vi "Main.vi"() -> ()   [LabVIEW 2017]
doc: "The myRIO Project template acquires acceleration data from the onboard accelerometer and displays the changes of acceleration values in a waveform chart."
uses:
  Y Axis Motor Cluster.ctl
  X Axis Motor Cluster.ctl
  Coords Input Cluster.ctl
  Motor Status Enum.ctl
  Encoder Cluster.ctl
  <vilib>/myRIO/Common/Instrument Driver Framework/myRIO v1.0/Encoder/typedefs/Encoder Count Direction Enum.ctl
  Motion Type Def.ctl
  <vilib>/myRIO/Instrument Drivers/Onboard IO/PWM/typedefs/PWM Reference.ctl
  <vilib>/myRIO/Common/Instrument Driver Framework/Utilities/typedefs/myRIO Generic Hardware Reference.ctl
  <vilib>/myRIO/Common/Instrument Driver Framework/Utilities/typedefs/Hardware Version Enum.ctl
  <vilib>/myRIO/Common/Instrument Driver Framework/Utilities/typedefs/myRIO v1.0 Reference.ctl
  <vilib>/myRIO/Common/Instrument Driver Framework/Utilities/typedefs/Generic FPGA Reference.ctl
  <vilib>/myRIO/Common/Instrument Driver Framework/myRIO v1.0/PWM/typedefs/PWM Channels Enum.ctl
  <vilib>/myRIO/Instrument Drivers/Onboard IO/PWM/typedefs/PWM Configuration.ctl
  <vilib>/userdefined/High Color/nirio_resource_hc.ctl
  <vilib>/myRIO/Common/Instrument Driver Framework/Utilities/vis/Is FPGA Ref Available.vi
  <vilib>/myRIO/Common/Instrument Driver Framework/myRIO v1.0/PWM/vis/myRIO v1.1 Open PWM.vi
  <vilib>/myRIO/Instrument Drivers/Onboard IO/PWM/vis/Set Duty Cycle and Frequency.vi
  <vilib>/myRIO/Common/Instrument Driver Framework/Utilities/vis/Validate Channels.vi
  <vilib>/myRIO/Common/Instrument Driver Framework/myRIO v1.0/PWM/vis/myRIO v1.0 Reserve PWM.vi
  <vilib>/myRIO/Common/Instrument Driver Framework/myRIO v1.0/UART/vis/myRIO v1.0 Close UART.vi
  <vilib>/myRIO/Common/Instrument Driver Framework/myRIO v1.0/PWM/vis/myRIO v1.0 Build MUX Configuration PWM.vi
  <vilib>/myRIO/Common/Instrument Driver Framework/myRIO v1.0/Resource Manager/vis/myRIO v1.0 Reserve Channel List.vi
  <vilib>/myRIO/Common/Instrument Driver Framework/myRIO v1.0/Resource Manager/vis/myRIO v1.0 Create Configuration List.vi
  <vilib>/myRIO/Common/Instrument Driver Framework/myRIO v1.0/Resource Manager/vis/myRIO v1.0 Reserve Channel.vi
  <vilib>/myRIO/Common/Instrument Driver Framework/myRIO v1.0/Resource Manager/vis/myRIO v1.0 Unreserve Channel.vi
  <vilib>/myRIO/Common/Instrument Driver Framework/myRIO v1.0/Resource Manager/vis/myRIO v1.0 Build Mutex Name.vi
  <vilib>/Utility/VariantDataType/GetNumericInfo.vi
  <vilib>/Utility/error.llb/Error Cluster From Error Code.vi
  <vilib>/myRIO/Common/Instrument Driver Framework/myRIO v1.0/myRIO v1.1 Open.vi
  <vilib>/myRIO/Common/Instrument Driver Framework/Utilities/vis/IO Manager.vi
  <vilib>/myRIO/Common/Instrument Driver Framework/Utilities/vis/Configuration Manager.vi
  <vilib>/myRIO/Common/Instrument Driver Framework/myRIO v1.0/Resource Manager/vis/myRIO v1.0 Configure IO.vi
  <vilib>/myRIO/Common/Instrument Driver Framework/myRIO v1.0/myRIO v1.0 Close.vi
  <vilib>/myRIO/Common/Instrument Driver Framework/myRIO v1.0/PWM/vis/myRIO v1.0 Write PWM.vi
  <vilib>/myRIO/Common/Instrument Driver Framework/Utilities/vis/FPGA Ref Manager.vi
  <vilib>/myRIO/Common/Instrument Driver Framework/myRIO v1.0/myRIO v1.0 Reset FPGA.vi
  <vilib>/myRIO/Common/Instrument Driver Framework/myRIO v1.0/IRQ/vis/myRIO v1.0 IRQ Info FGV.vi
  <vilib>/myRIO/Common/Instrument Driver Framework/myRIO v1.0/IRQ/vis/myRIO v1.0 Timer IRQ Info FGV.vi
  <vilib>/myRIO/Common/Instrument Driver Framework/myRIO v1.0/IRQ/vis/myRIO v1.0 ISR Agent.vi
  <vilib>/myRIO/Express VI/Onboard IO/PWM/PWM Express VI.xnode
  <vilib>/myRIO/Instrument Drivers/Onboard IO/PWM/vis/myRIO PWM Open.xnode
  <vilib>/myRIO/Instrument Drivers/Utilities/Utilities.lvlib
  <vilib>/myRIO/Instrument Drivers/Onboard IO/PWM/PWM.lvlib
panel:
  out "Motion Planning Outputs":T1
  in  "Motion Planning Inputs":T2
  out "Motion Profile":T3=enum."Triangular"
  out "Converted\nPWM Frequency":dbl
  out "Encoder Output":T4
  out "X Axis state":T6
  out "Y Axis state":T6
  out "Loop Runtime (s)":dbl format="%.3f"
  in  "Clear Chart History":bool
  in  "Coordinates Input":T7
  out "Y Axis":T8(graph)
  out "X Axis":T8(graph)
  in  "X Axis Motor Target":T9
  out "X Axis Motor Params":T10
  in  "Y Axis Setpoint":T11
  out "Y Axis Motor Params":T12
  in  "stop":bool
  out "Total Runtime (s)":dbl format="%.2f"
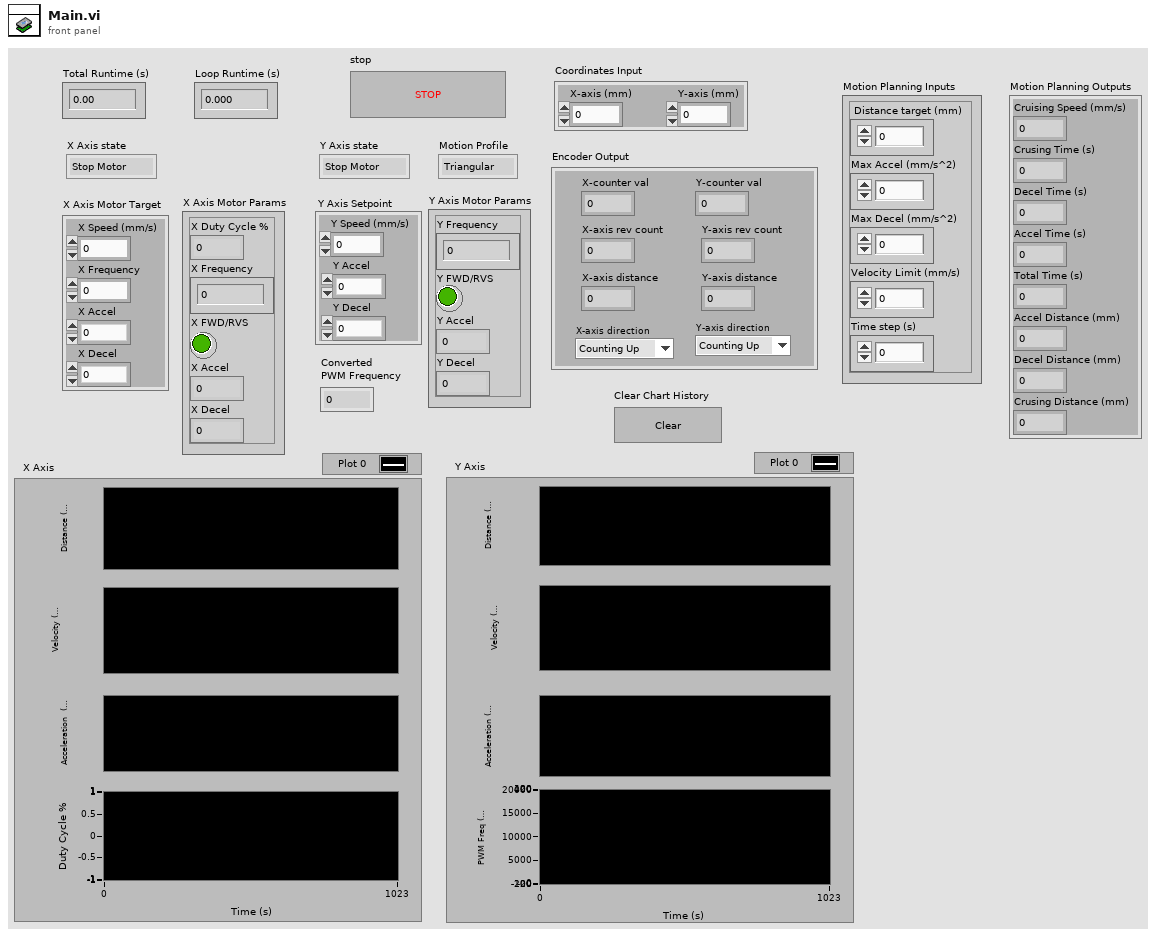
[diagram p1: front panel]
types:
  T1 = cluster{"Cruising Speed (mm/s)":dbl, "Crusing Time (s)":dbl, "Decel Time (s)":dbl, "Accel Time (s)":dbl, "Total Time (s)":dbl, "Accel Distance (mm)":dbl, "Decel Distance (mm)":dbl, "Crusing Distance (mm)":dbl}
  T2 = cluster{" Distance target (mm)":dbl, "Max Accel (mm/s^2)":dbl, "Max Decel (mm/s^2)":dbl, "Velocity Limit (mm/s) ":dbl, "Time step (s)":dbl}
  T3 = typedef "Motion Type Def.ctl" = enum16{"Trapezodial", "Triangular"}
  T4 = typedef "Encoder Cluster.ctl" = cluster{"Y-axis rev count":dbl, "Y-axis distance":dbl, "X-axis rev count":dbl, "X-axis distance":dbl, "Y-axis direction":T5, "X-axis direction":T5, "X-counter val":i32, "Y-counter val":i32}
  T5 = typedef "Encoder Count Direction Enum.ctl" = enum16{"Counting Up", "Counting Down"}
  T6 = typedef "Motor Status Enum.ctl" = enum16{"Stop Motor", "Read Inputs", "Steady Speed", "Accelerate", "Decelerate"}
  T7 = typedef "Coords Input Cluster.ctl" = cluster{"X-axis (mm)":dbl, "Y-axis (mm)":dbl}
  T8 = cluster{"X-axis distance":dbl, dbl, dbl, "X Frequency":dbl}
  T9 = cluster{"X Frequency":dbl, "X Accel":dbl, "X Decel":dbl, "X Speed (mm/s)":dbl}
  T10 = typedef "X Axis Motor Cluster.ctl" = cluster{"X Frequency":dbl, "X FWD/RVS":bool, "X Accel":dbl, "X Decel":dbl, "X Duty Cycle %":dbl}
  T11 = cluster{"Y Speed (mm/s)":dbl, "Y Accel":dbl, "Y Decel":dbl}
  T12 = typedef "Y Axis Motor Cluster.ctl" = cluster{"Y Frequency":dbl, "Y FWD/RVS":bool, "Y Accel":dbl, "Y Decel":dbl}
  T13 = cluster{"X Frequency":dbl, "X FWD/RVS":bool, "X Accel":dbl, "X Decel":dbl, "X Duty Cycle %":dbl}
  T14 = cluster{"Y Frequency":dbl, "Y FWD/RVS":bool, "Y Accel":dbl, "Y Decel":dbl}
  T15 = cluster{"X-axis distance":dbl, dbl, dbl, "X Frequency":dbl}[]
  T16 = enum16{"800", "1600", "3200", "6400", "12800", "25600"}
  T17 = cluster{"Y-axis distance":dbl, dbl, dbl, "Y Frequency":dbl}
  T18 = cluster{"X-axis rev count":dbl, dbl, dbl, "X Duty Cycle %":dbl}
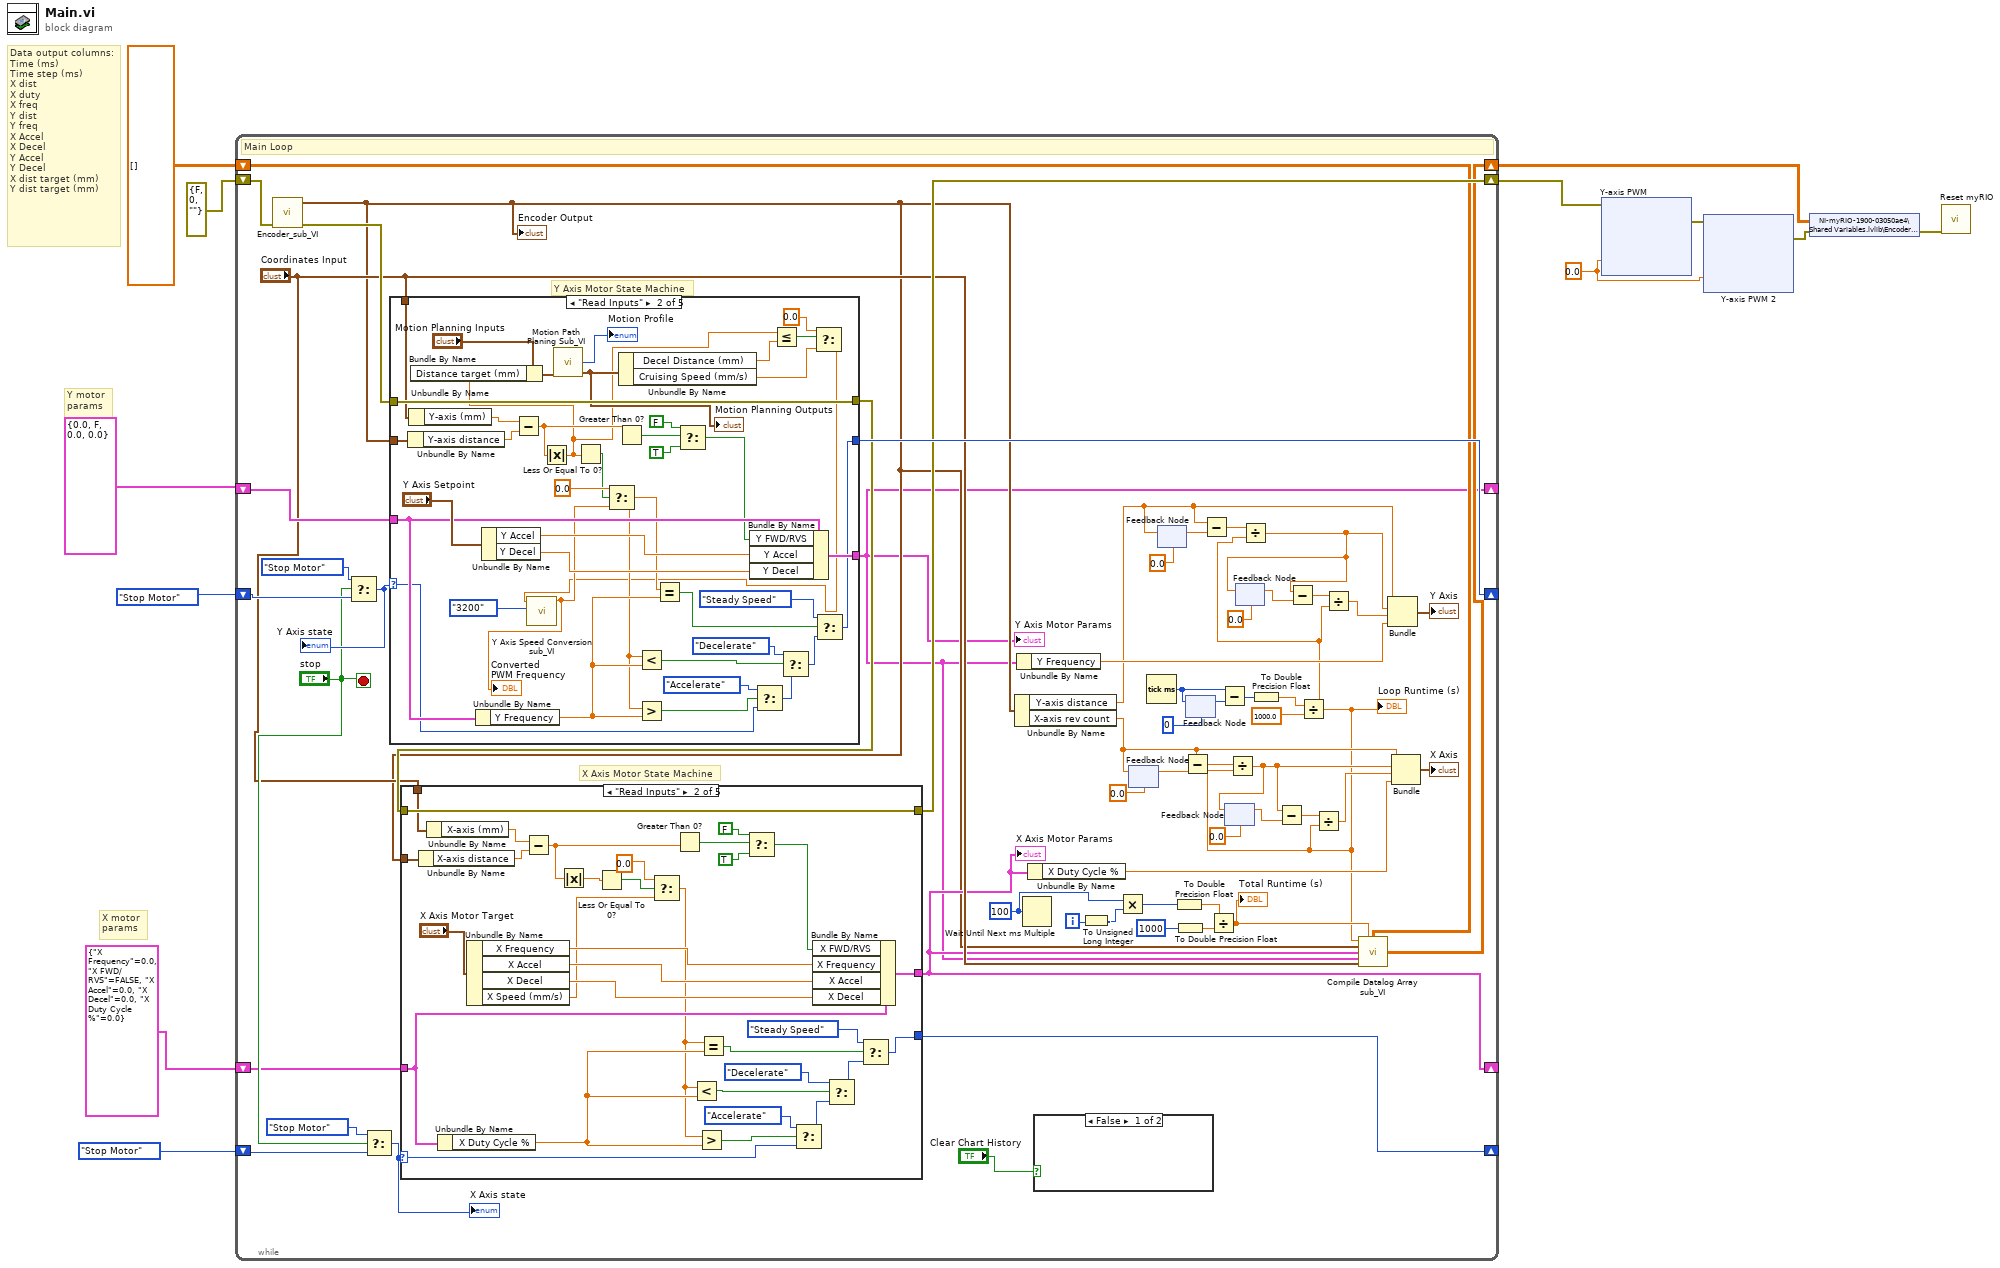
[diagram p0: block diagram]
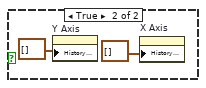
[diagram p2: hidden frame]
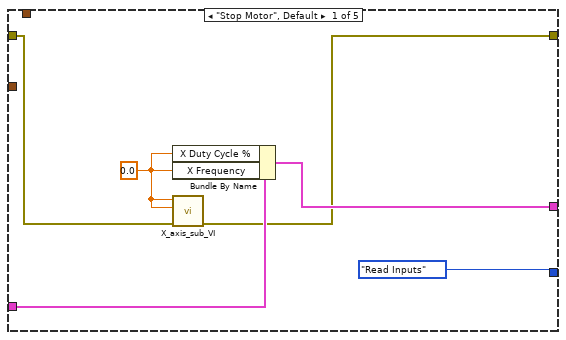
[diagram p3: hidden frame]
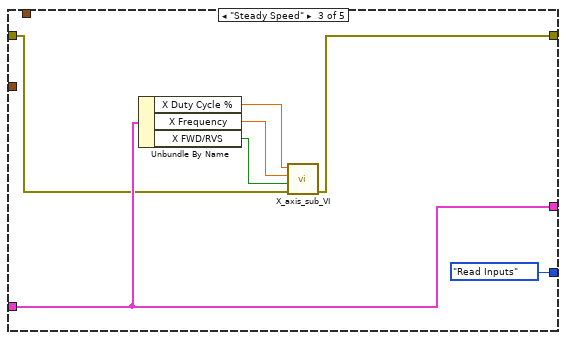
[diagram p4: hidden frame]
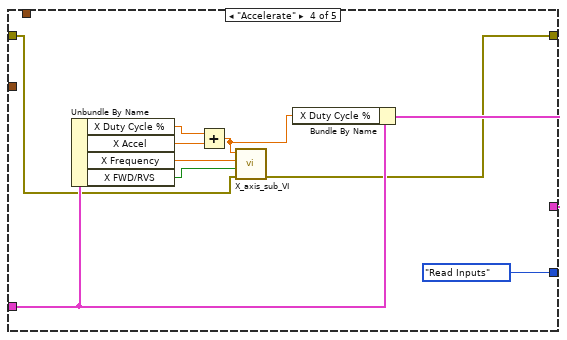
[diagram p5: hidden frame]
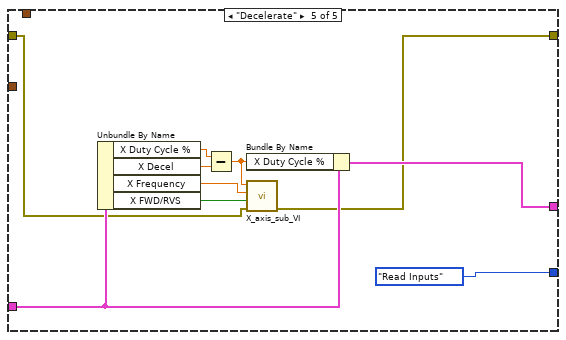
[diagram p6: hidden frame]
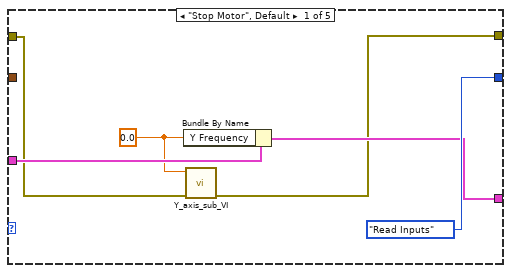
[diagram p7: hidden frame]
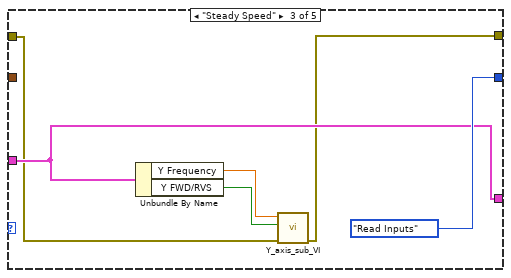
[diagram p8: hidden frame]
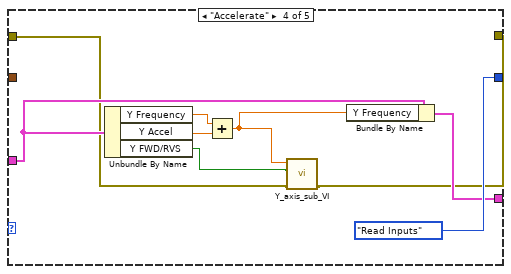
[diagram p9: hidden frame]
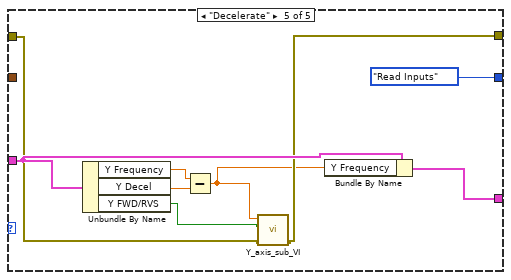
[diagram p10: hidden frame]
diagram:
  w6 = 0.0 ("Frequency [Hz]")
  # "X motor \nparams"
  # "Y motor \nparams"
  # "Data output columns:\nTime (ms)\nTime step (ms)\nX dist\nX duty\nX freq\nY dist\nY freq\nX Accel\nX Decel\nY Accel\nY Decel\nX dist target (mm)\nY dist target (mm)"
  n1 = while {
    shift-right: [w57] -> w12
    shift-left: errorcluster {"status"=FALSE, "code"=0, "source"=""} ("error in (no error)") -> [w71]
    shift-right: [w39] -> w1
    shift-left: dbl[][] [] -> [w40]
    shift-right: [w32] -> _
    shift-left: T14 {"Y Frequency"=0.0, "Y FWD/RVS"=FALSE, "Y Accel"=0.0, "Y Decel"=0.0} ("Y Axis Motor Params 2") -> [w70]
    shift-right: [w69] -> _
    shift-left: Motor_Status_Enum."Stop Motor" -> [w67]
    shift-right: [w60] -> _
    shift-left: Motor_Status_Enum."Stop Motor" -> [w62]
    shift-right: [w36] -> _
    shift-left: T13 {"X Frequency"=0.0, "X FWD/RVS"=FALSE, "X Accel"=0.0, "X Decel"=0.0, "X Duty Cycle %"=0.0} ("X Axis Motor Params 3") -> [w59]
    i -> [w46]
    stop <- "stop" stop-if-true
    w45 = u32 100 ("milliseconds to wait")
    # "X Axis Motor State Machine"
    # "Y Axis Motor State Machine"
    # "Main Loop"
    n2 = call "Encoder_sub_VI.vi"("error in (no error)"=w71) -> ("error out"=w65:errorcluster, "Encoder Output"=w33:T4)  [unwired: 9 in]
    "Encoder Output" <- w33
    n3 = Select(t=Motor_Status_Enum."Stop Motor", s="stop", f=w67) -> (s? t:f=w68:T6)
    "Y Axis state" <- w68
    n4 = Select(t=Motor_Status_Enum."Stop Motor", s="stop", f=w62) -> (s? t:f=w63:T6)
    "X Axis state" <- w63
    n5 = case shown="\"Read Inputs\"" w68 {
      selector: w68 -> [_ w171 _ _ _]
      tunnel: w70 -> [w144 w172 w188 w197 w205]
      tunnel: [Motor_Status_Enum."Read Inputs" w161 Motor_Status_Enum."Read Inputs" Motor_Status_Enum."Read Inputs" Motor_Status_Enum."Read Inputs"] -> w69
      tunnel: [w142 w173 w188 w196 w206] -> w32
      tunnel: w65 -> [w140 w170 w187 w193 w203]
      tunnel: [w141 w170 w186 w192 w204] -> w58
      tunnel: w33 -> [_ w169 _ _ _]
      tunnel: "Coordinates Input" -> [_ w165 _ _ _]
      frame "Stop Motor", Default {
        w139 = 0.0 ("Y Frequency")
        n6 = Bundle By Name(cluster=w144, "Y Frequency"=w139) -> (w142:T14)
        n7 = call "Y_axis_sub_VI.vi"("error in (no error)"=w140, "Frequency"=w139) -> ("error out"=w141:errorcluster)  [unwired: 9 in]
      }
      frame "Read Inputs" {
        n8 = Unbundle By Name(w169) -> ("Y-axis distance"=w157:dbl)
        n9 = Unbundle By Name(w165) -> ("Y-axis (mm)"=w158:dbl)
        n10 = Unbundle By Name(w172) -> ("Y Frequency"=w179:dbl)
        n11 = Unbundle By Name("Y Axis Setpoint") -> ("Y Accel"=w183:dbl, "Y Decel"=w184:dbl)
        n12 = Subtract(x=w158, y=w157) -> (x-y=w152:dbl)
        n13 = Absolute Value(x=w152) -> (abs(x)=w145:dbl)
        n14 = Bundle By Name(cluster="Motion Planning Inputs", "Distance target (mm)"=w145) -> (w155:T2)
        n15 = call "Motion Path Planing Sub_VI.vi"("Motion Planning Inputs"=w155) -> ("Motion Profile"=→"Motion Profile":T3, "Motion Planning Outputs"=w153:T1)  [unwired: 4 in, 1 out]
        "Motion Planning Outputs" <- w153
        n16 = Less Or Equal To 0?(x=w145) -> (x <= 0?=w156:bool)
        n17 = Greater Than 0?(x=w152) -> (x > 0?=w164:bool)
        n18 = Unbundle By Name(w153) -> ("Decel Distance (mm)"=w151:dbl, "Cruising Speed (mm/s)"=w147:dbl)
        n19 = Select(t=FALSE, s=w164, f=TRUE) -> (s? t:f=w166:bool)
        n20 = Bundle By Name(cluster=w172, "Y FWD/RVS"=w166, "Y Accel"=w183, "Y Decel"=w184) -> (w173:T14)
        n21 = Less Or Equal?(x=w145, y=w151) -> (x <= y?=w150:bool)
        n22 = Select(t=0.0, s=w150, f=w147) -> (s? t:f=w148:dbl)
        n23 = call "Y Axis Speed Conversion sub_VI.vi"("Microsteps per Rev"=T16."3200", "Setpoint\nSpeed (mm/s)"=w148) -> ("PWM Frequency"=w160:dbl)  [unwired: 9 in]
        "Converted\nPWM Frequency" <- w160
        n24 = Select(t=0.0, s=w156, f=w160) -> (s? t:f=w162:dbl)
        n25 = Less?(x=w162, y=w179) -> (x < y?=w176:bool)
        n26 = Greater?(x=w162, y=w179) -> (0:w185:bool)
        n27 = Equal?(x=w162, y=w179) -> (x = y?=w180:bool)
        n28 = Select(t=Motor_Status_Enum."Accelerate", s=w185, f=w171) -> (s? t:f=w178:T6)
        n29 = Select(t=Motor_Status_Enum."Decelerate", s=w176, f=w178) -> (s? t:f=w181:T6)
        n30 = Select(t=Motor_Status_Enum."Steady Speed", s=w180, f=w181) -> (s? t:f=w161:T6)
      }
      frame "Steady Speed" {
        n31 = Unbundle By Name(w188) -> ("Y Frequency"=w190:dbl, "Y FWD/RVS"=w191:bool)
        n32 = call "Y_axis_sub_VI.vi"("error in (no error)"=w187, "FWD/RVS"=w191, "Frequency"=w190) -> ("error out"=w186:errorcluster)  [unwired: 8 in]
      }
      frame "Accelerate" {
        n33 = Unbundle By Name(w197) -> ("Y Frequency"=w199:dbl, "Y Accel"=w200:dbl, "Y FWD/RVS"=w194:bool)
        n34 = Add(x=w199, y=w200) -> (x+y=w195:dbl)
        n35 = call "Y_axis_sub_VI.vi"("error in (no error)"=w193, "FWD/RVS"=w194, "Frequency"=w195) -> ("error out"=w192:errorcluster)  [unwired: 8 in]
        n36 = Bundle By Name(cluster=w197, "Y Frequency"=w195) -> (w196:T14)
      }
      frame "Decelerate" {
        n37 = Unbundle By Name(w205) -> ("Y Frequency"=w209:dbl, "Y Decel"=w208:dbl, "Y FWD/RVS"=w202:bool)
        n38 = Subtract(x=w209, y=w208) -> (x-y=w201:dbl)
        n39 = call "Y_axis_sub_VI.vi"("error in (no error)"=w203, "FWD/RVS"=w202, "Frequency"=w201) -> ("error out"=w204:errorcluster)  [unwired: 8 in]
        n40 = Bundle By Name(cluster=w205, "Y Frequency"=w201) -> (w206:T14)
      }
    }
    "Y Axis Motor Params" <- w32
    n41 = case shown="\"Read Inputs\"" w63 {
      selector: w63 -> [_ w99 _ _ _]
      tunnel: [Motor_Status_Enum."Read Inputs" w92 Motor_Status_Enum."Read Inputs" Motor_Status_Enum."Read Inputs" Motor_Status_Enum."Read Inputs"] -> w60
      tunnel: [w76 w98 w115 w122 w132] -> w36
      tunnel: w59 -> [w77 w97 w115 w121 w131]
      tunnel: w58 -> [w75 w95 w113 w120 w130]
      tunnel: [w74 w95 w112 w119 w129] -> w57
      tunnel: w33 -> [_ w94 _ _ _]
      tunnel: "Coordinates Input" -> [_ w93 _ _ _]
      frame "Stop Motor", Default {
        w79 = 0.0 ("Y Frequency")
        n42 = Bundle By Name(cluster=w77, "X Duty Cycle %"=w79, "X Frequency"=w79) -> (w76:T13)
        n43 = call "X_axis_sub_VI.vi"("error in (no error)"=w75, "Frequency"=w79, "Duty Cycle %"=w79) -> ("error out"=w74:errorcluster)  [unwired: 8 in]
      }
      frame "Read Inputs" {
        n44 = Unbundle By Name(w94) -> ("X-axis distance"=w83:dbl)
        n45 = Unbundle By Name(w93) -> ("X-axis (mm)"=w84:dbl)
        n46 = Unbundle By Name(w97) -> ("X Duty Cycle %"=w110:dbl)
        n47 = Unbundle By Name("X Axis Motor Target") -> ("X Frequency"=w102:dbl, "X Accel"=w100:dbl, "X Decel"=w101:dbl, "X Speed (mm/s)"=w88:dbl)
        n48 = Subtract(x=w84, y=w83) -> (x-y=w80:dbl)
        n49 = Absolute Value(x=w80) -> (abs(x)=w81:dbl)
        n50 = Less Or Equal To 0?(x=w81) -> (x <= 0?=w82:bool)
        n51 = Select(t=0.0, s=w82, f=w88) -> (s? t:f=w87:dbl)
        n52 = Greater Than 0?(x=w80) -> (x > 0?=w90:bool)
        n53 = Less?(x=w87, y=w110) -> (x < y?=w105:bool)
        n54 = Greater?(x=w87, y=w110) -> (0:w103:bool)
        n55 = Equal?(x=w87, y=w110) -> (x = y?=w109:bool)
        n56 = Select(t=FALSE, s=w90, f=TRUE) -> (s? t:f=w85:bool)
        n57 = Select(t=Motor_Status_Enum."Accelerate", s=w103, f=w99) -> (s? t:f=w107:T6)
        n58 = Bundle By Name(cluster=w97, "X FWD/RVS"=w85, "X Frequency"=w102, "X Accel"=w100, "X Decel"=w101) -> (w98:T13)
        n59 = Select(t=Motor_Status_Enum."Decelerate", s=w105, f=w107) -> (s? t:f=w108:T6)
        n60 = Select(t=Motor_Status_Enum."Steady Speed", s=w109, f=w108) -> (s? t:f=w92:T6)
      }
      frame "Steady Speed" {
        n61 = Unbundle By Name(w115) -> ("X Duty Cycle %"=w117:dbl, "X Frequency"=w116:dbl, "X FWD/RVS"=w118:bool)
        n62 = call "X_axis_sub_VI.vi"("error in (no error)"=w113, "FWD/RVS"=w118, "Frequency"=w116, "Duty Cycle %"=w117) -> ("error out"=w112:errorcluster)  [unwired: 7 in]
      }
      frame "Accelerate" {
        n63 = Unbundle By Name(w121) -> ("X Duty Cycle %"=w124:dbl, "X Accel"=w125:dbl, "X Frequency"=w126:dbl, "X FWD/RVS"=w128:bool)
        n64 = Add(x=w124, y=w125) -> (x+y=w127:dbl)
        n65 = call "X_axis_sub_VI.vi"("error in (no error)"=w120, "FWD/RVS"=w128, "Frequency"=w126, "Duty Cycle %"=w127) -> ("error out"=w119:errorcluster)  [unwired: 7 in]
        n66 = Bundle By Name(cluster=w121, "X Duty Cycle %"=w127) -> (w122:T13)
      }
      frame "Decelerate" {
        n67 = Unbundle By Name(w131) -> ("X Duty Cycle %"=w134:dbl, "X Decel"=w135:dbl, "X Frequency"=w136:dbl, "X FWD/RVS"=w138:bool)
        n68 = Subtract(x=w134, y=w135) -> (x-y=w137:dbl)
        n69 = Bundle By Name(cluster=w131, "X Duty Cycle %"=w137) -> (w132:T13)
        n70 = call "X_axis_sub_VI.vi"("error in (no error)"=w130, "FWD/RVS"=w138, "Frequency"=w136, "Duty Cycle %"=w137) -> ("error out"=w129:errorcluster)  [unwired: 7 in]
      }
    }
    "X Axis Motor Params" <- w36
    n71 = Unbundle By Name(w33) -> ("Y-axis distance"=w30:dbl, "X-axis rev count"=w16:dbl)
    n72 = Unbundle By Name(w32) -> ("Y Frequency"=w34:dbl)
    n73 = Wait Until Next ms Multiple(millisecond multiple=w45) -> ()  [unwired: 1 out]
    n74 = Unbundle By Name(w36) -> ("X Duty Cycle %"=w35:dbl)
    n75 = case shown="False" "Clear Chart History" {
      frame False {
      }
      frame True {
        n76 = property on="Y Axis" class="WFChart (strict)"("History Data"=T15 []) -> ()  [unwired: 2 in, 2 out]
        n77 = property on="X Axis" class="WFChart (strict)"("History Data"=T15 []) -> ()  [unwired: 2 in, 2 out]
      }
    }
    n78 = To Unsigned Long Integer(number=w46) -> (unsigned 32bit integer=w44:u32)
    n79 = Multiply(x=w45, y=w44) -> (x*y=w43:u32)
    n80 = feedback #1(0.0) -> (w21:dbl)
    n81 = feedback-in #1(w16) -> ()
    n82 = Tick Count (ms)() -> (millisecond timer value=w49:u32)
    n83 = feedback #2(0.0) -> (w29:dbl)
    n84 = feedback-in #2(w30) -> ()
    n85 = To Double Precision Float(number=w43) -> (double precision float=w42:dbl)
    n86 = To Double Precision Float(number=u32 1000 ("y")) -> (double precision float=w41:dbl)
    n87 = Subtract(x=w16, y=w21) -> (x-y=w20:dbl)
    n88 = feedback-in #3(w49) -> ()
    n89 = feedback #3(u32 0) -> (w48:u32)
    n90 = Subtract(x=w30, y=w29) -> (x-y=w28:dbl)
    n91 = Divide(x=w42, y=w41) -> (x/y=w37:dbl)
    "Total Runtime (s)" <- w37
    n92 = Subtract(x=w49, y=w48) -> (x-y=w52:u32)
    n93 = feedback #4(0.0) -> (w18:dbl)
    n94 = feedback #5(0.0) -> (w26:dbl)
    n95 = To Double Precision Float(number=w52) -> (double precision float=w50:dbl)
    n96 = Divide(x=w50, y=1000.0) -> (x/y=w13:dbl)
    "Loop Runtime (s)" <- w13
    n97 = Divide(x=w20, y=w13) -> (x/y=w15:dbl)
    n98 = feedback-in #4(w15) -> ()
    n99 = Divide(x=w28, y=w13) -> (x/y=w25:dbl)
    n100 = feedback-in #5(w25) -> ()
    n101 = Subtract(x=w15, y=w18) -> (x-y=w17:dbl)
    n102 = Subtract(x=w25, y=w26) -> (x-y=w24:dbl)
    n103 = Divide(x=w17, y=w13) -> (x/y=w14:dbl)
    n104 = Divide(x=w24, y=w13) -> (x/y=w23:dbl)
    n105 = call "Compile Datalog Array sub_VI.vi"("Loop Runtime (s)"=w13, "Total Runtime (s)"=w37, "Initialised Array"=w40, "Encoder Output"=w33, "X Axis Motor Params"=w36, "Y Axis Motor Params"=w32, "Coordinates Input"="Coordinates Input") -> ("Data Array"=w39:dbl[][])  [unwired: 8 in]
    n106 = Bundle("Y-axis distance"=w30, w25, w23, "Y Frequency"=w34) -> (→"Y Axis":T17)  [unwired: 1 in]
    n107 = Bundle("X-axis rev count"=w16, w15, w14, "X Duty Cycle %"=w35) -> (→"X Axis":T18)  [unwired: 1 in]
  }
  n108 = xnode "Y-axis PWM"("Frequency [Hz]"=w6, "error in (no error)"=w12) -> ("error out"=w8:errorcluster)
  n109 = xnode "Y-axis PWM 2"("Frequency [Hz]"=w6, "error in (no error)"=w8) -> ("error out"=w7:errorcluster)
  n110 = shared-variable "NI-myRIO-1900-03050ae4\\Shared Variables.lvlib\\Encoder Data"(w1, error in=w7) -> (error out=w9:errorcluster)
  n111 = call <vilib>:"Reset myRIO.vi"("error in (no error)"=w9) -> ()  [unwired: 10 in, 1 out]
